vi "Update Results.vi"(8 "error in":errorcluster, 10 "measurement results":variant, 11 "measure call context in":refnum<class "Measure Call Context.lvclass">) -> (0 "error out":errorcluster, 3 "measure call context out":refnum<class "Measure Call Context.lvclass">)   [LabVIEW 2020, in "NI Measurement Plug-In SDK.lvlib" / "Measure Call Context.lvclass"]
doc: "Sends measurement updates to a measurement client, like InstrumentStudio. Do not use this VI to write the final results. Instead, use the Measurement Results indicator of the Measurement Logic VI to write the final measurement result.\n\nThis VI must be called with the Measurement Results cluster as the input. You must always update all elements of the cluster, including unchanged values.\n\nInstrumentStudio does not cache data from previous updates so you must write all of the data to the cluster to display cumulative updates.\n\nTestStand gnores updates from this VI and only uses the final measurement result."
uses:
  Measure Call Context.lvclass
  Measure Call Context.lvclass/Measure Call Context.ctl
  IMeasurement Service/IMeasurement Service.lvclass
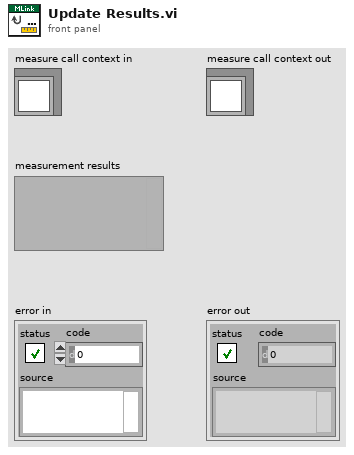
[diagram p1: front panel]
types:
  T1 = typedef "NI Measurement Plug-In SDK.lvlib/Measure Call Context.lvclass/Data.ctl" = cluster{"pin map context":T2, "gRPC ID":T3, "measurement service":refnum<class "IMeasurement Service.lvclass">, "measurement plugin service":refnum<class "Measurement Plugin Service.lvclass">, "reserved session infos":set{T4}}
  T2 = typedef "NI Measurement Plug-In SDK.lvlib/Pin Map Context.ctl" = cluster{"pin map id":string, "sites":i32[]}
  T3 = typedef "grpc-lvsupport-release.lvlib/grpcId.ctl" = u64
  T4 = typedef "ni.measurementlink.sessionmanagement.v1.api.lvlib/ni_measurementlink_sessionmanagement_v1_SessionInformation.ctl" = cluster{"session":T5, "resource_name":string, "channel_list":string, "instrument_type_id":string, "session_exists":bool, "channel_mappings":T6[]}
  T5 = typedef "ni.measurementlink.sessionmanagement.v1.api.lvlib/nidevice_grpc_Session.ctl" = cluster{"name":string}
  T6 = typedef "ni.measurementlink.sessionmanagement.v1.api.lvlib/ni_measurementlink_sessionmanagement_v1_ChannelMapping.ctl" = cluster{"pin_or_relay_name":string, "site":i32, "channel":string, "multiplexer_resource_name":string, "multiplexer_route":string}
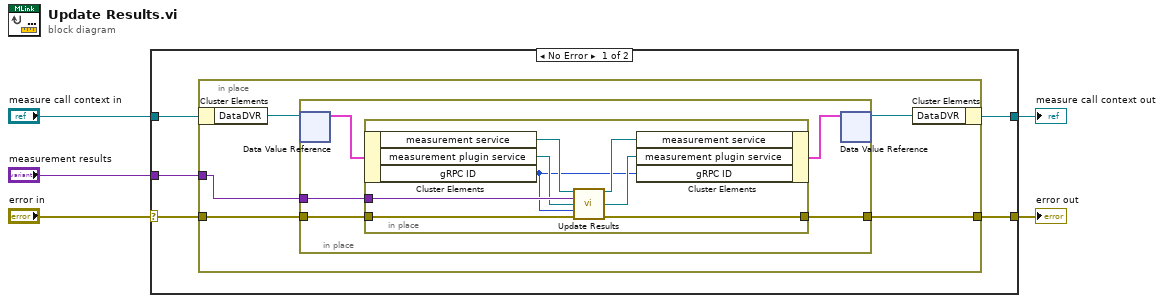
[diagram p0: block diagram]
diagram:
  n1 = case shown="No Error" "error in" {
    selector: "error in" -> [w8 w30]
    tunnel: [w7 w30] -> w4
    tunnel: [w6 w29] -> w2
    tunnel: "measure call context in" -> [w10 w29]
    tunnel: "measurement results" -> [w9 _]
    frame No Error {
      n2 = in-place {
        in-place-border: w9 -> [w15]
        in-place-border: w8 -> [w14]
        in-place-border: [w13] -> w7
        n3 = in-place-cluster #1(w10) -> ("DataDVR"=w12:refnum<data-value>)
        n4 = in-place {
          in-place-border: w15 -> [w20]
          in-place-border: w14 -> [w19]
          in-place-border: [w18] -> w13
          n5 = in-place-dvr #2(w12) -> (w17:T1)  [unwired: 1 out]
          n6 = in-place {
            in-place-border: w20 -> [w28]
            in-place-border: w19 -> [w27]
            in-place-border: [w26] -> w18
            n7 = in-place-cluster #3(w17) -> ("measurement service"=w25:refnum<class "IMeasurement Service.lvclass">, "measurement plugin service"=w24:refnum<class "Measurement Plugin Service.lvclass">, "gRPC ID"=w21:T3)
            n8 = call-dynamic "Update Results.vi"("measurement service in"=w25, "measurement results"=w28, "measurement plugin service in"=w24, "gRPC ID in"=w21, "error in"=w27) -> ("measurement service out"=w23:refnum<class "IMeasurement Service.lvclass">, "measurement plugin service out"=w22:refnum<class "Measurement Plugin Service.lvclass">, "error out"=w26:errorcluster)  [unwired: 8 in]
            n9 = in-place-cluster #3("measurement service"=w23, "measurement plugin service"=w22, "gRPC ID"=w21) -> (w16:T1)
          }
          n10 = in-place-dvr #2(w16) -> (w11:refnum<data-value>)  [unwired: 1 out]
        }
        n11 = in-place-cluster #1("DataDVR"=w11) -> (w6:refnum<class "Measure Call Context.lvclass">)
      }
    }
    frame Error {
    }
  }
  "error out" <- w4
  "measure call context out" <- w2
